vi "DangerEnemy.vi"(10 "IA Input":T1={"our_robots"=[], "enemy_robots"=[], "balls"=[], "geometry"={"line_width"=0, "field_length"=0, "field_width"=0, "boundary_width"=0, "referee_width"=0, "goal_width"=0, "goal_depth"=0, "goal_wall_width"=0, "center_circle_radius"=0, "defense_radius"=0, "defense_stretch"=0, "free_kick_from_defense_dist"=0, "penalty_spot_from_field_line_dist"=0, "penalty_line_from_spot_dist"=0}, "IA Judge"={"stage"="", "command"="", "our_goalie_id"=0.0, "enemy_goalie_id"=0.0, "command enum"=enum."Halt", "Time"=enum."Azul"}, "Received Timestamp"=timestamp(0 s since 1904-01-01), "Events"={"Touch"=FALSE, "Ball out"=FALSE, "id touch"=0.0, "Ball out of \nVision"=FALSE, "Ball inside \nGoalie area"=FALSE, "Robot not responding"=FALSE, "Robots responding status"=[1.0, 1.0, 1.0, 1.0, 1.0, 1.0], "Enemy Ball \nPossession"=FALSE, "Pass State"=FALSE, "id end of pass"=0.0, "Kick"=FALSE, "Id ini Possession"=0.0, "Ball Possesion"=FALSE, "Id Possesion"=0.0, "Direct Kick"=FALSE, "2nd Strk Ativo"=FALSE}}) -> (0 "Pos do segundo inimigo\nperigoso":dbl[](array[numeric]), 1 "id do segundo inimigo\nmais perigoso":i32, 2 "Pos do inimigo\nperigoso":dbl[](array[numeric]), 3 "id do inimigo\nmais perigoso":u32, 4 "Id do Inimigo Mais Próximo":u32, 5 "Numero de inimigos\npossiveis para marcar":i32)   [LabVIEW 2022 SP3]
uses:
  <vilib>/Analysis/NI_AALPro.lvlib
  <vilib>/Analysis/_algsub.llb/Real Vector Norm.vi
  Controls/Functions Enum.ctl
  Controls/AttackerStates.ctl
  Controls/AI Robot.ctl
  Controls/AI Ball.ctl
  Controls/Field Size.ctl
  Controls/Command Enum.ctl
  Controls/AI Judge.ctl
  Controls/Events.ctl
  Controls/AI Input.ctl
  Controls/PathDest.ctl
  Controls/PathDests.ctl
panel:
  in  "D para nao marcar":dbl=200.0
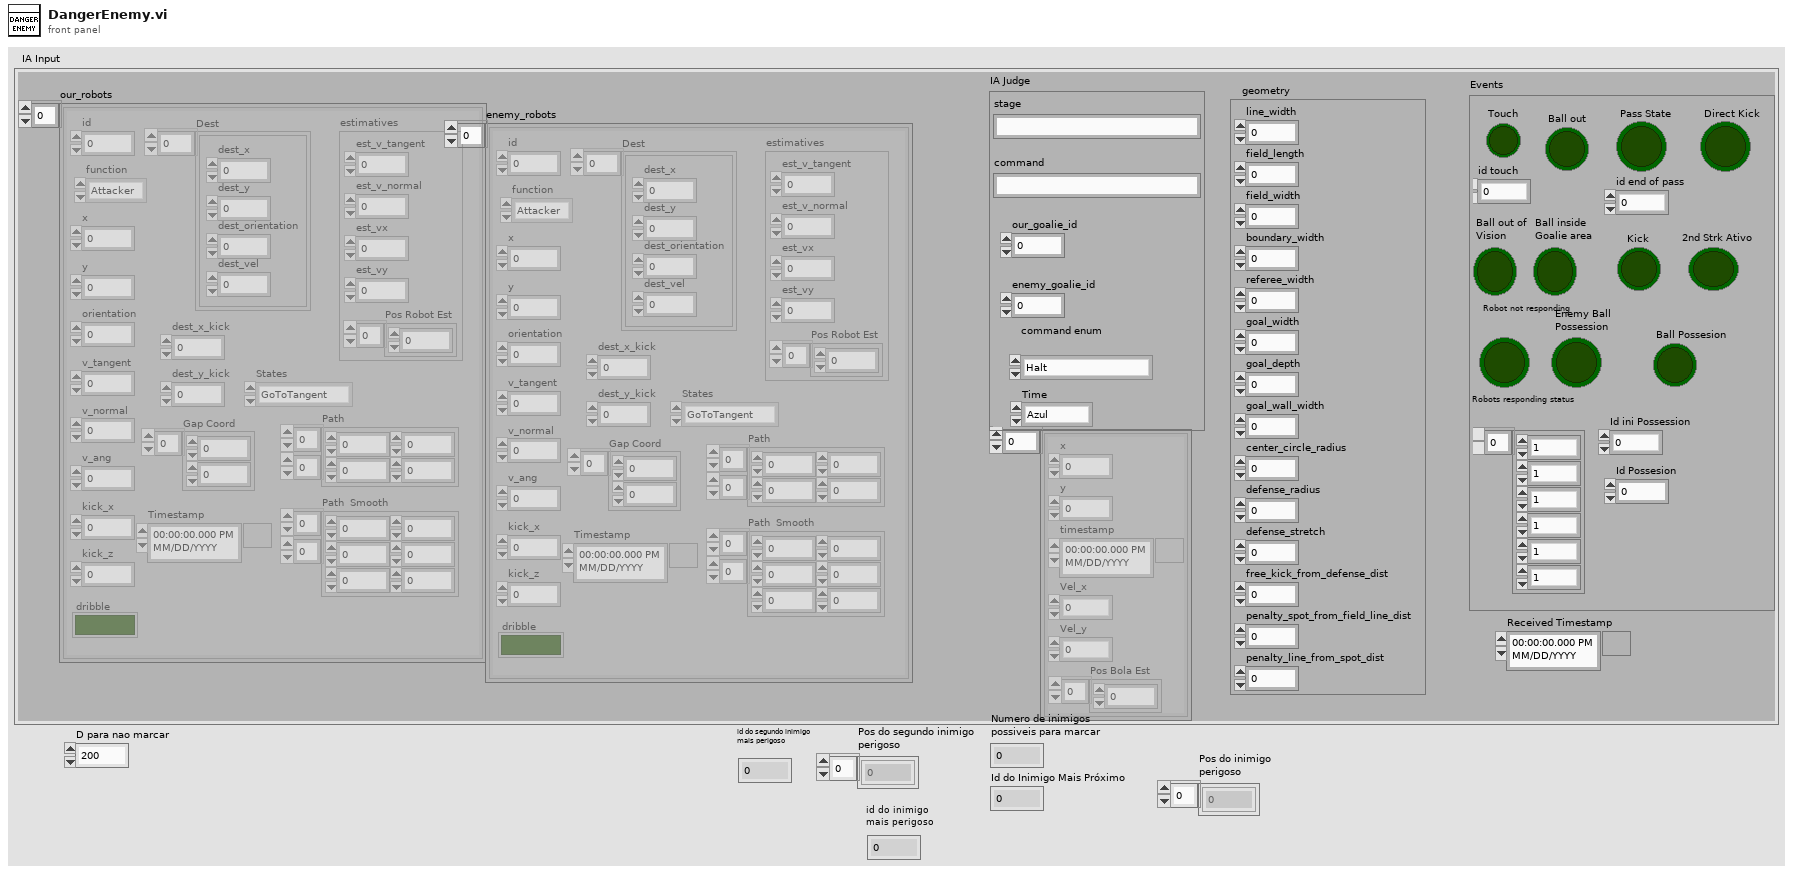
[diagram p1: front panel]
types:
  T1 = typedef "AI Input.ctl" = cluster{"our_robots":T2[], "enemy_robots":T2[], "balls":T7[], "geometry":T8, "IA Judge":T9, "Received Timestamp":timestamp, "Events":T11}
  T2 = typedef "AI Robot.ctl" = cluster{"id":u32, "function":T3, "x":dbl, "y":dbl, "orientation":dbl, "v_tangent":dbl, "v_normal":dbl, "v_ang":dbl, "kick_x":dbl, "kick_z":dbl, "dribble":bool, "Timestamp":timestamp, "estimatives":cluster{"est_v_tangent":dbl, "est_v_normal":dbl, "est_vx":dbl, "est_vy":dbl, "Pos Robot Est":dbl[]}, "dest_x_kick":dbl, "dest_y_kick":dbl, "Gap Coord":dbl[], "States":T4, "Path ":dbl[][], "Path  Smooth":dbl[][], "Dest":T5}
  T3 = typedef "Functions Enum.ctl" = enum16{"2nd Striker", "Attacker", "Goalie", "Defender", "Striker", "Goto 0", "Dummy", "Kicker", "ZigZag 0", "ZigZag 1", "ZigZag 2", "ZigZag 3", "ZigZag 4", "ZigZag 5", "ZigZag 6", "ZigZag 7", "ZigZag 8", ""}
  T4 = typedef "AttackerStates.ctl" = enum16{"Pass", "GoToTangent", "BallGetting", "GoToKick", ""}
  T5 = typedef "PathDests.ctl" = T6[]
  T6 = typedef "PathDest.ctl" = cluster{"dest_x":dbl, "dest_y":dbl, "dest_orientation":dbl, "dest_vel":dbl}
  T7 = typedef "AI Ball.ctl" = cluster{"x":dbl, "y":dbl, "timestamp":timestamp, "Vel_x":dbl, "Vel_y":dbl, "Pos Bola Est":dbl[]}
  T8 = typedef "Field Size.ctl" = cluster{"line_width":u32, "field_length":u32, "field_width":u32, "boundary_width":u32, "referee_width":u32, "goal_width":u32, "goal_depth":u32, "goal_wall_width":u32, "center_circle_radius":u32, "defense_radius":u32, "defense_stretch":u32, "free_kick_from_defense_dist":u32, "penalty_spot_from_field_line_dist":u32, "penalty_line_from_spot_dist":u32}
  T9 = typedef "AI Judge.ctl" = cluster{"stage":string, "command":string, "our_goalie_id":dbl, "enemy_goalie_id":dbl, "command enum":T10, "Time":enum16{"Azul", "Amarelo"}}
  T10 = typedef "Command Enum.ctl" = enum16{"Halt", "Stop", "Force Start", "PKA Normal Start", "Prepare Kickoff Ally", "PKE Normal Start", "Prepare Kickoff Enemy", "Prepare Penalty Ally", "PPA Normal Start", "Prepare Penalty Enemy", "PPE Normal Start", "Direct Free Enemy", "Direct Free Ally", "Indirect Free Enemy", "Indirect Free Ally", "Timeout Enemy", "Timeout Ally", "Goal Enemy", "Goal Ally", "Ball Placement Enemy", "Ball Placement Ally", "Normal Half Time", "Extra Time Break", "Extra Half Time", "None", "Post Game"}
  T11 = typedef "Events.ctl" = cluster{"Touch":bool, "Ball out":bool, "id touch":dbl, "Ball out of \nVision":bool, "Ball inside \nGoalie area":bool, "Robot not responding":bool, "Robots responding status":dbl[], "Enemy Ball \nPossession":bool, "Pass State":bool, "id end of pass":dbl, "Kick":bool, "Id ini Possession":dbl, "Ball Possesion":bool, "Id Possesion":dbl, "Direct Kick":bool, "2nd Strk Ativo":bool}
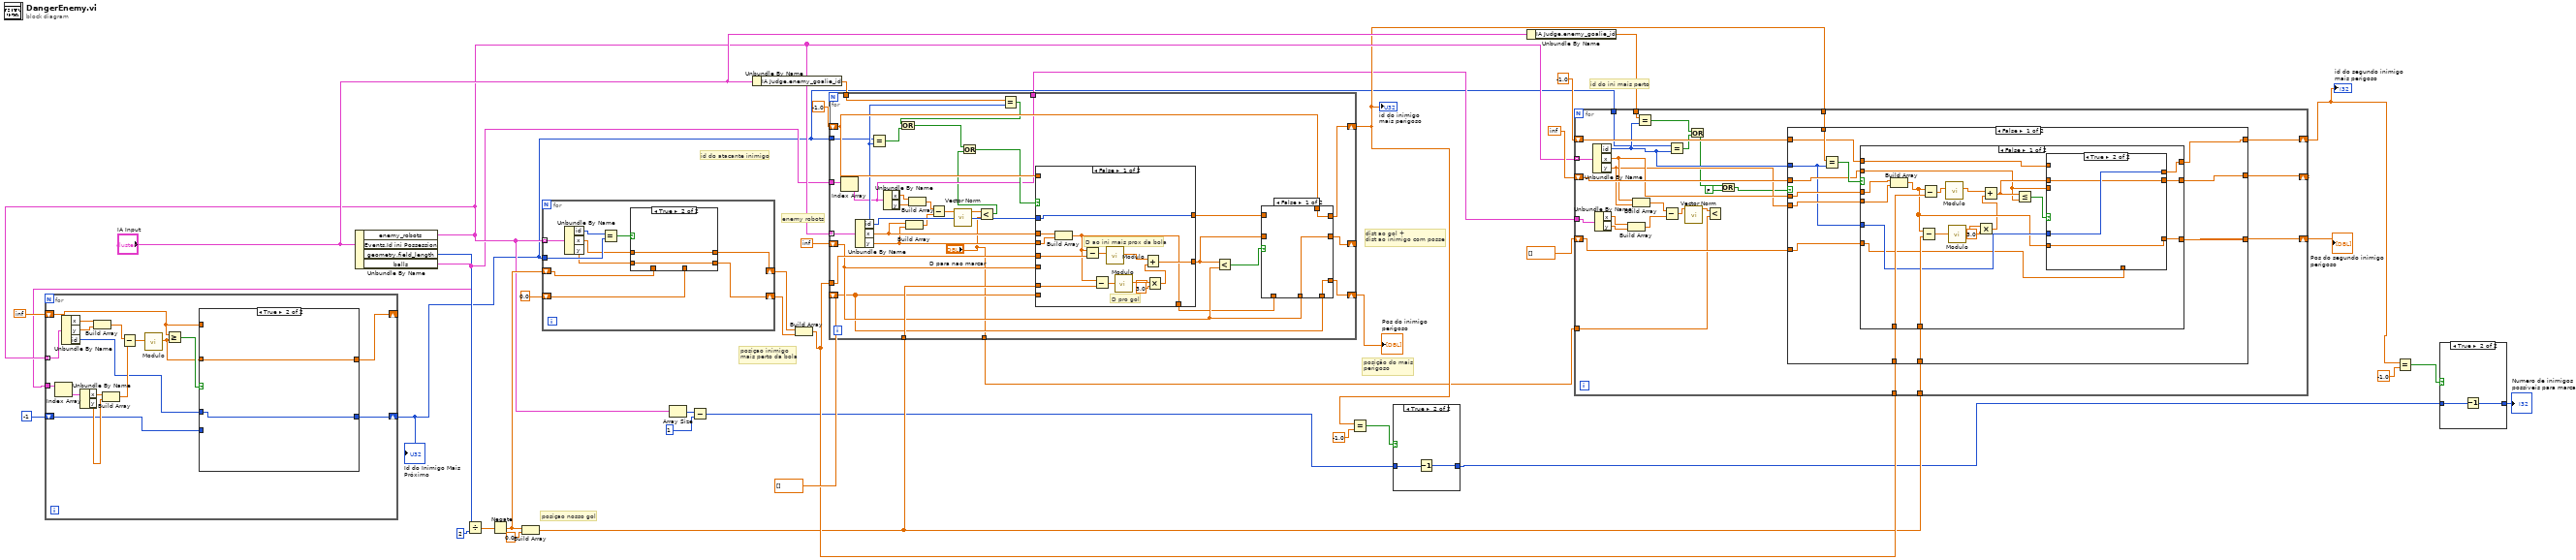
[diagram p0: block diagram]
diagram:
  # "id do ini mais perto"
  # "id do atacante inimigo"
  # "enemy robots"
  # "dist ao gol +\ndist ao inimigo com posse"
  # "posição do mais\nperigoso"
  # "posiçao nosso gol"
  # "posiçao inimigo\nmais perto da bola"
  n1 = Unbundle By Name("IA Input") -> ("enemy_robots"=w19:T2[], "geometry.field_length"=w38:u32, "balls"=w7:T7[])  [unwired: 1 out]
  n2 = for {
    tunnel: w19 -> [w56] mode=indexing
    tunnel: w7 -> [w55]
    shift-right: [w44] -> _
    shift-left: inf -> [w41]
    shift-right: [w42] -> w2
    shift-left: -1 -> [w40]
    n3 = Index Array(array=w55) -> (element=w54:T7)  [unwired: 1 in]
    n4 = Unbundle By Name(w56) -> ("x"=w53:dbl, "y"=w52:dbl, "id"=w43:u32)
    n5 = Unbundle By Name(w54) -> ("x"=w51:dbl, "y"=w50:dbl)
    n6 = Build Array(w53, w52) -> (w49:dbl[])
    n7 = Build Array(w51, w50) -> (w48:dbl[])
    n8 = Subtract(x=w49, y=w48) -> (x-y=w46:dbl[])
    n9 = call "Modulo.vi"("2D vector"=w46) -> ("Modulo"=w45:dbl)  [unwired: 10 in]
    n10 = Greater Or Equal?(x=w41, y=w45) -> (x >= y?=w47:bool)
    n11 = case shown="True" w47 {
      tunnel: [w58 w60] -> w44
      tunnel: w45 -> [_ w60]
      tunnel: w43 -> [_ w59]
      tunnel: [w57 w59] -> w42
      tunnel: w41 -> [w58 _]
      tunnel: w40 -> [w57 _]
      frame False {
      }
      frame True {
      }
    }
  }
  "Id do Inimigo Mais Próximo" <- w2
  n12 = Divide(x=w38, y=u32 2) -> (x/y=w36:dbl)
  n13 = Negate(x=w36) -> (-x=w31:dbl)
  n14 = Build Array(w31, 0.0 ("element")) -> (w25:dbl[])
  n15 = for {
    tunnel: w19 -> [w70] mode=indexing
    tunnel: w2 -> [w69]
    shift-right: [w64] -> w4
    shift-left: w31 -> [w62]
    shift-right: [w63] -> w39
    shift-left: 0.0 ("y") -> [w61]
    n16 = Unbundle By Name(w70) -> ("id"=w67:u32, "x"=w66:dbl, "y"=w65:dbl)
    n17 = Equal?(x=w67, y=w69) -> (x = y?=w68:bool)
    n18 = case shown="True" w68 {
      tunnel: w66 -> [_ w74]
      tunnel: w65 -> [_ w73]
      tunnel: [w72 w74] -> w64
      tunnel: [w71 w73] -> w63
      tunnel: w62 -> [w72 _]
      tunnel: w61 -> [w71 _]
      frame False {
      }
      frame True {
      }
    }
  }
  n19 = Array Size(array=w19) -> (size(s)=w18:i32)
  n20 = Subtract(x=w18, y=1) -> (x-y=w13:i32)
  n21 = Unbundle By Name("IA Input") -> ("IA Judge.enemy_goalie_id"=w22:dbl)
  n22 = Build Array(w4, w39) -> (w26:dbl[])
  n23 = for {
    tunnel: w19 -> [w106] mode=indexing
    tunnel: w26 -> [w105]
    tunnel: w25 -> [w104]
    shift-right: [w101] -> _
    shift-left: inf -> [w100]
    shift-right: [w98] -> w16
    shift-left: -1.0 ("id") -> [w95]
    shift-right: [w96] -> w34
    shift-left: dbl[] [] -> [w94]
    tunnel: w22 -> [w93]
    tunnel: w7 -> [w89]
    tunnel: [w78] -> w6
    tunnel: ["D para nao marcar"] -> w5
    tunnel: w2 -> [w76]
    n24 = Index Array(array=w89) -> (element=w78:T7)  [unwired: 1 in]
    n25 = Unbundle By Name(w106) -> ("id"=w92:u32, "x"=w86:dbl, "y"=w85:dbl)
    n26 = Equal?(x=w76, y=w92) -> (x = y?=w90:bool)
    n27 = Unbundle By Name(w78) -> ("x"=w88:dbl, "y"=w87:dbl)
    n28 = Build Array(w86, w85) -> (w83:dbl[])
    n29 = Build Array(w88, w87) -> (w84:dbl[])
    n30 = Subtract(x=w84, y=w83) -> (x-y=w82:dbl[])
    n31 = call-poly <vilib>:"Vector Norm.vi"("Input Vector"=w82) -> ("norm"=w81:dbl)  [unwired: 9 in, 1 out]
    n32 = Less?(x=w81, y="D para nao marcar") -> (x < y?=w75:bool)
    n33 = Equal?(x=w93, y=w92) -> (x = y?=w91:bool)
    n34 = Or(x=w91, y=w90) -> (x .or. y?=w80:bool)
    n35 = Or(x=w80, y=w75) -> (x .or. y?=w79:bool)
    n36 = case shown="False" w79 {
      tunnel: w86 -> [w125 _]
      tunnel: w85 -> [w124 _]
      tunnel: w105 -> [w123 _]
      tunnel: w104 -> [w121 _]
      tunnel: [w118 w128] -> w102
      tunnel: w100 -> [_ w128]
      tunnel: w92 -> [w117 _]
      tunnel: [w117 w127] -> w99
      tunnel: [w116 w126] -> w97
      tunnel: w95 -> [_ w127]
      tunnel: w94 -> [_ w126]
      frame False {
        # "D ao ini mais prox da bola"
        # "D pro gol"
        n37 = Build Array(w125, w124) -> (w116:dbl[])
        n38 = Subtract(x=w116, y=w123) -> (x-y=w122:dbl[])
        n39 = Subtract(x=w116, y=w121) -> (x-y=w120:dbl[])
        n40 = call "Modulo.vi"("2D vector"=w122) -> ("Modulo"=w119:dbl)  [unwired: 10 in]
        n41 = call "Modulo.vi"("2D vector"=w120) -> ("Modulo"=w115:dbl)  [unwired: 10 in]
        n42 = Multiply(x=w115, y=3.0) -> (x*y=w113:dbl)
        n43 = Add(x=w119, y=w113) -> (x+y=w118:dbl)
      }
      frame True {
      }
    }
    n44 = Less?(x=w102, y=w100) -> (x < y?=w103:bool)
    n45 = case shown="False" w103 {
      tunnel: w102 -> [_ w112]
      tunnel: [w109 w112] -> w101
      tunnel: w100 -> [w109 _]
      tunnel: [w108 w111] -> w98
      tunnel: w99 -> [_ w111]
      tunnel: w95 -> [w108 _]
      tunnel: w97 -> [_ w110]
      tunnel: [w107 w110] -> w96
      tunnel: w94 -> [w107 _]
      frame False {
      }
      frame True {
        # "mais perigoso"
      }
    }
  }
  "id do inimigo\nmais perigoso" <- w16
  "Pos do inimigo\nperigoso" <- w34
  n46 = Equal?(x=w16, y=-1.0) -> (x = y?=w14:bool)
  n47 = case shown="True" w14 {
    tunnel: w13 -> [w129 w131]
    tunnel: [w129 w130] -> w9
    frame False {
    }
    frame True {
      n48 = Decrement(x=w131) -> (x-1=w130:i32)
    }
  }
  n49 = Unbundle By Name("IA Input") -> ("IA Judge.enemy_goalie_id"=w20:dbl)
  n50 = for {
    tunnel: w19 -> [w159] mode=indexing
    shift-right: [w158] -> w11
    shift-left: -1.0 -> [w157]
    shift-right: [w156] -> _
    shift-left: inf -> [w150]
    shift-right: [w155] -> w27
    shift-left: dbl[] [] -> [w154]
    tunnel: w16 -> [w153]
    tunnel: w26 -> [w152]
    tunnel: w25 -> [w151]
    tunnel: w20 -> [w149]
    tunnel: w6 -> [w143]
    tunnel: w5 -> [w136]
    tunnel: w2 -> [w133]
    n51 = Unbundle By Name(w159) -> ("id"=w148:u32, "x"=w145:dbl, "y"=w144:dbl)
    n52 = Unbundle By Name(w143) -> ("x"=w142:dbl, "y"=w141:dbl)
    n53 = Build Array(w142, w141) -> (w139:dbl[])
    n54 = Build Array(w145, w144) -> (w140:dbl[])
    n55 = Equal?(x=w149, y=w148) -> (x = y?=w147:bool)
    n56 = Subtract(x=w140, y=w139) -> (x-y=w138:dbl[])
    n57 = Equal?(x=w133, y=w148) -> (x = y?=w146:bool)
    n58 = call-poly <vilib>:"Vector Norm.vi"("Input Vector"=w138) -> ("norm"=w137:dbl)  [unwired: 9 in, 1 out]
    n59 = Or(x=w147, y=w146) -> (x .or. y?=w135:bool)
    n60 = Less?(x=w137, y=w136) -> ()  [unwired: 1 out]
    n61 = Or(x=w135, y=FALSE) -> (x .or. y?=w134:bool)
    n62 = case shown="False" w134 {
      tunnel: w157 -> [w170 w204]
      tunnel: [w169 w204] -> w158
      tunnel: w150 -> [w168 w203]
      tunnel: [w167 w203] -> w156
      tunnel: w154 -> [w166 w202]
      tunnel: [w165 w202] -> w155
      tunnel: w148 -> [w160 _]
      tunnel: w153 -> [w172 _]
      tunnel: w145 -> [w164 _]
      tunnel: w144 -> [w163 _]
      tunnel: w152 -> [w162 _]
      tunnel: w151 -> [w161 _]
      frame False {
        n63 = Equal?(x=w172, y=w160) -> (x = y?=w171:bool)
        n64 = case shown="False" w171 {
          tunnel: [w184 w201] -> w169
          tunnel: w170 -> [w182 w201]
          tunnel: w168 -> [w176 w200]
          tunnel: [w180 w200] -> w167
          tunnel: w166 -> [w177 w199]
          tunnel: [w178 w199] -> w165
          tunnel: w164 -> [w192 _]
          tunnel: w163 -> [w191 _]
          tunnel: w162 -> [w190 _]
          tunnel: w161 -> [w187 _]
          tunnel: w160 -> [w183 _]
          frame False {
            n65 = Build Array(w192, w191) -> (w179:dbl[])
            n66 = Subtract(x=w179, y=w187) -> (x-y=w186:dbl[])
            n67 = Subtract(x=w179, y=w190) -> (x-y=w189:dbl[])
            n68 = call "Modulo.vi"("2D vector"=w189) -> ("Modulo"=w188:dbl)  [unwired: 10 in]
            n69 = call "Modulo.vi"("2D vector"=w186) -> ("Modulo"=w175:dbl)  [unwired: 10 in]
            n70 = Multiply(x=w175, y=3.0) -> (x*y=w173:dbl)
            n71 = Add(x=w188, y=w173) -> (x+y=w181:dbl)
            n72 = Less Or Equal?(x=w181, y=w176) -> (x <= y?=w185:bool)
            n73 = case shown="True" w185 {
              tunnel: [w195 w198] -> w184
              tunnel: w183 -> [_ w198]
              tunnel: w182 -> [w195 _]
              tunnel: [w193 w197] -> w180
              tunnel: w181 -> [_ w197]
              tunnel: [w194 w196] -> w178
              tunnel: w179 -> [_ w196]
              tunnel: w177 -> [w194 _]
              tunnel: w176 -> [w193 _]
              frame False {
              }
              frame True {
              }
            }
          }
          frame True {
          }
        }
      }
      frame True {
      }
    }
  }
  "id do segundo inimigo\nmais perigoso" <- w11
  "Pos do segundo inimigo\nperigoso" <- w27
  n74 = Equal?(x=w11, y=-1.0) -> (x = y?=w10:bool)
  n75 = case shown="True" w10 {
    tunnel: w9 -> [w205 w207]
    tunnel: [w205 w206] -> w8
    frame False {
    }
    frame True {
      n76 = Decrement(x=w207) -> (x-1=w206:i32)
    }
  }
  "Numero de inimigos\npossiveis para marcar" <- w8
